vi "get_user_comments.vi"(8 "error in (no error)":errorcluster, 9 "string in":string, 11 "ErrorController in":refnum<class "ErrorController.lvclass">) -> (0 "error out":errorcluster, 1 "string out":string, 2 "user comments":string, 3 "ErrorController out":refnum<class "ErrorController.lvclass">)   [LabVIEW 2010, in "ErrorController.lvclass"]
uses:
  ErrorController.lvclass
  ErrorController.lvclass/ErrorController.ctl
  <vilib>/Utility/file.llb/Read From Spreadsheet File (string).vi
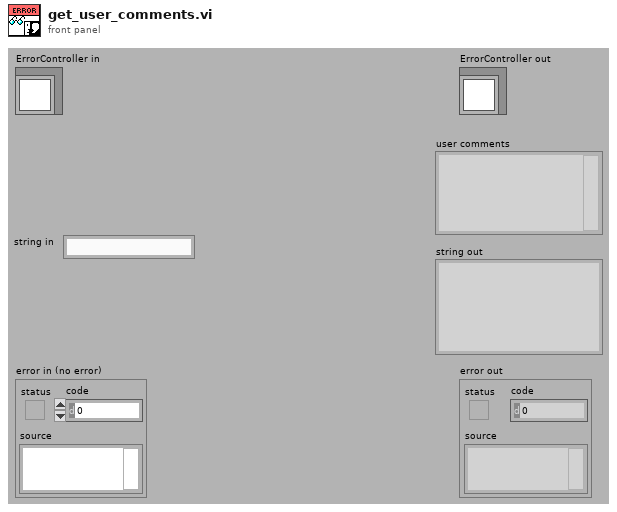
[diagram p1: front panel]
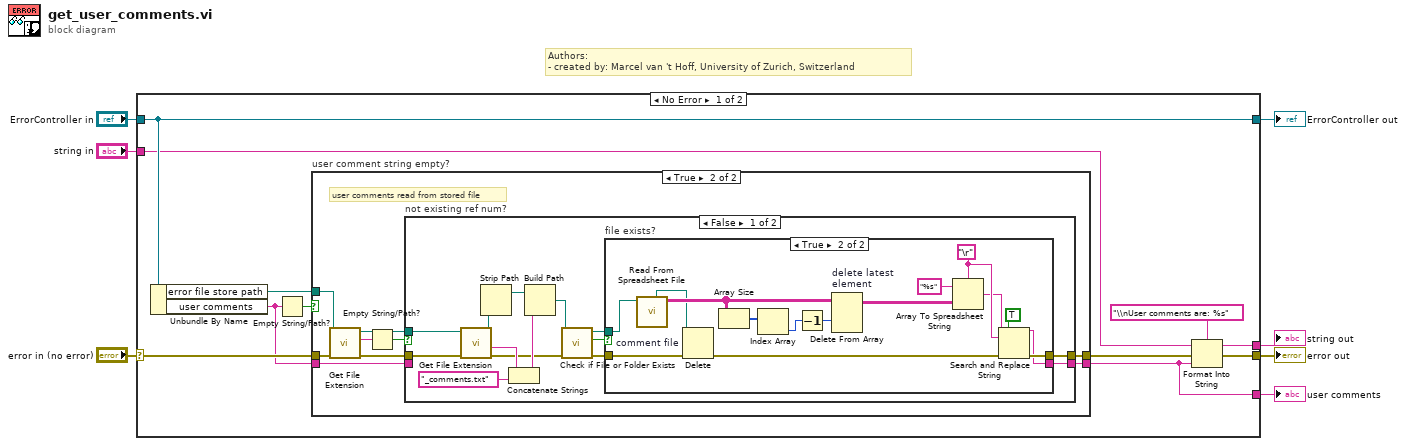
[diagram p0: block diagram]
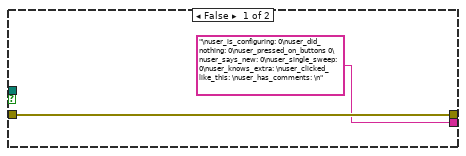
[diagram p3: hidden frame]
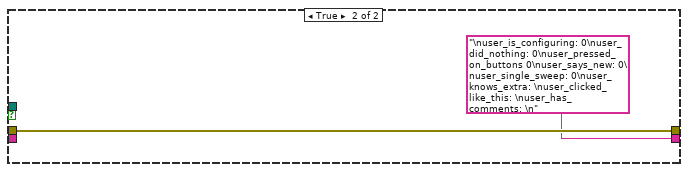
[diagram p4: hidden frame]
diagram:
  # "Authors: \n- created by: Marcel van 't Hoff, University of Zurich, Switzerland"
  n1 = case shown="No Error" "error in (no error)" {
    selector: "error in (no error)" -> [w13 w64]
    tunnel: [w14 w64] -> w6
    tunnel: [w18 w63] -> w4
    tunnel: "ErrorController in" -> [w18 w63]
    tunnel: [w10 _] -> w1
    tunnel: "string in" -> [w17 _]
    tunnel: [w16 _] -> w2
    frame No Error {
      n2 = Unbundle By Name(w18) -> ("error file store path"=w9:path, "user comments"=w11:string)
      n3 = Empty String/Path?(string/path=w11) -> (empty?=w8:bool)
      n4 = case "user comment string empty?" shown="True" w8 {
        tunnel: w13 -> [w20 w26]
        tunnel: [w20 w27] -> w12
        tunnel: [w19 w29] -> w10
        tunnel: w11 -> [w19 w21]
        tunnel: w9 -> [_ w24]
        frame False {
          # "comment read out from private data"
        }
        frame True {
          # "user comments read from stored file"
          n5 = call <vilib>:"Get File Extension.vi"("error in (no error)"=w26, "file"=w24) -> ("error out"=w25:errorcluster, "lowercase file extension"=w22:string, "dup file"=w23:path)  [unwired: 6 in, 1 out]
          n6 = Empty String/Path?(string/path=w22) -> (empty?=w28:bool)
          n7 = case "not existing ref num?" shown="False" w28 {
            tunnel: [w35 "\nuser_is_configuring: 0\nuser_did_nothing: 0\nuser_pressed_on_buttons 0\nuser_says_new: 0\nuser_single_sweep: 0\nuser_knows_extra: \nuser_clicked_like_this: \nuser_has_comments: \n" ("string out")] -> w29
            tunnel: w23 -> [w38 _]
            tunnel: w25 -> [w37 w62]
            tunnel: [w36 w62] -> w27
            tunnel: w21 -> [_ _]
            frame False {
              n8 = call <vilib>:"Get File Extension.vi"("error in (no error)"=w37, "file"=w38) -> ("error out"=w34:errorcluster, "filename without extension"=w40:string, "dup file"=w39:path)  [unwired: 6 in, 1 out]
              n9 = Strip Path(path=w39) -> (stripped path=w42:path)  [unwired: 1 out]
              n10 = Concatenate Strings(w40, "_comments.txt" ("string")) -> (w43:string)
              n11 = Build Path(base path=w42, name or relative path=w43) -> (appended path=w32:path)
              n12 = call <vilib>:"Check if File or Folder Exists.vi"("error in (no error)"=w34, "path"=w32) -> ("error out"=w33:errorcluster, "file or folder exists?"=w30:bool, "dup path"=w31:path)  [unwired: 7 in]
              n13 = case "file exists?" shown="True" w30 {
                tunnel: [w45 w58] -> w36
                tunnel: ["\nuser_is_configuring: 0\nuser_did_nothing: 0\nuser_pressed_on_buttons 0\nuser_says_new: 0\nuser_single_sweep: 0\nuser_knows_extra: \nuser_clicked_like_this: \nuser_has_comments: \n" ("string out") w55] -> w35
                tunnel: w33 -> [w45 w47]
                tunnel: w31 -> [_ w46]
                frame False {
                }
                frame True {
                  w57 = "\r"
                  n14 = call-poly <vilib>:"Read From Spreadsheet File.vi"("file path (dialog if empty)"=w46) -> ("all rows"=w49:string[][], "new file path (Not A Path if cancelled)"=w48:path)  [unwired: 6 in, 3 out]
                  n15 = Delete "comment file"(path (use dialog)=w48, error in=w47) -> (error out=w50:errorcluster)  [unwired: 3 in, 2 out]
                  n16 = Array Size(array=w49) -> (size(s)=w54:i32[])
                  n17 = Index Array(array=w54) -> (element=w53:i32)  [unwired: 1 in]
                  n18 = Decrement(x=w53) -> (x-1=w51:i32)
                  n19 = Delete From Array "delete latest\nelement"(array=w49, index (row)=w51) -> (array with subset deleted=w52:string[][])  [unwired: 2 in, 1 out]
                  n20 = Array To Spreadsheet String(delimiter (Tab)=w57, array=w52, 3:"%s" ("format string")) -> (spreadsheet string=w56:string)
                  n21 = Search and Replace String(replace all?=TRUE ("replace all? (F)"), input string=w56, search string=w57, error in=w50) -> (result string=w55:string, error out=w58:errorcluster)  [unwired: 4 in, 2 out]
                }
              }
            }
            frame True {
            }
          }
        }
      }
      n22 = Format Into String(format string="\\nUser comments are: %s", initial string=w17, error in=w12, w10) -> (resulting string=w16:string, error out=w14:errorcluster)
    }
    frame Error {
    }
  }
  "error out" <- w6
  "ErrorController out" <- w4
  "user comments" <- w1
  "string out" <- w2
